vi "Datos de la grafica.vi"(7 "Tipo de señal":T1(ring), 8 "error in (no error)":errorcluster, 9 "Amplitud":dbl, 10 "frecuencia":dbl, 11 "GUI SeñalActualizable in":refnum<class "GUI SeñalActualizable.lvclass">) -> (0 "error out":errorcluster, 3 "GUI SeñalActualizable out":refnum<class "GUI SeñalActualizable.lvclass">)   [LabVIEW 2020, in "GUI SeñalActualizable.lvlib" / "GUI SeñalActualizable.lvclass"]
uses:
  <vilib>/measure/NI_MABase.lvlib
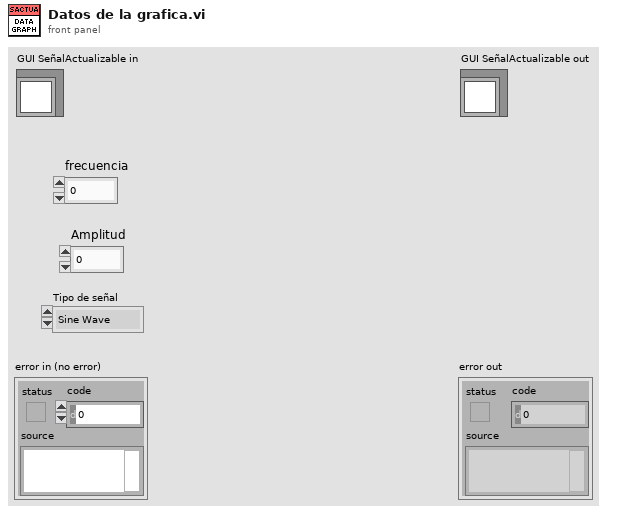
[diagram p1: front panel]
types:
  T1 = enum16{"Sine Wave", "Triangle Wave", "Square Wave", "Sawtooth Wave"}
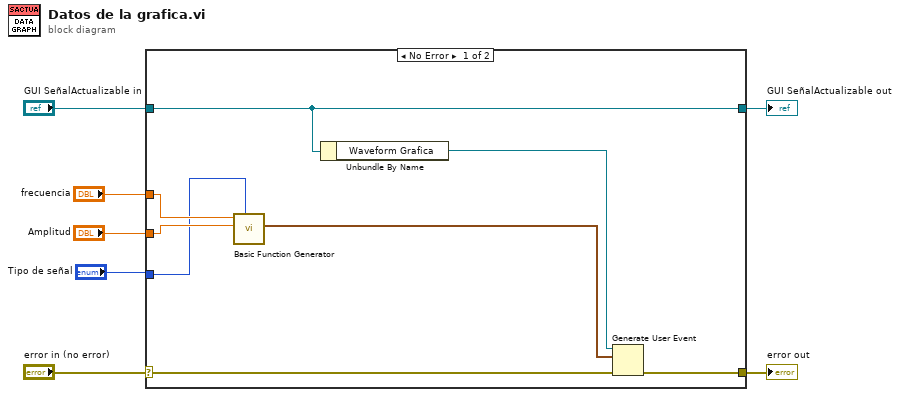
[diagram p0: block diagram]
diagram:
  n1 = case shown="No Error" "error in (no error)" {
    selector: "error in (no error)" -> [w10 w17]
    tunnel: [w11 w17] -> w6
    tunnel: [w12 w16] -> w4
    tunnel: "GUI SeñalActualizable in" -> [w12 w16]
    tunnel: "Tipo de señal" -> [w13 _]
    tunnel: "Amplitud" -> [w15 _]
    tunnel: "frecuencia" -> [w14 _]
    frame No Error {
      n2 = call <vilib>:"Basic Function Generator.vi"("signal type"=w13, "amplitude"=w15, "frequency"=w14) -> ("signal out"=w8:waveform(dbl))  [unwired: 6 in, 2 out]
      n3 = Unbundle By Name(w12) -> ("Waveform Grafica"=w9:refnum<user-event>)
      n4 = Generate User Event(user event=w9, event data cluster=w8, error in=w10) -> (error out=w11:errorcluster)  [unwired: 1 in, 1 out]
    }
    frame Error {
    }
  }
  "error out" <- w6
  "GUI SeñalActualizable out" <- w4
